vi "Read Pulsed Voltage.vi"(0 "VISA resource name":refnum<visa-resource-name>, 1 "Pulse Off Time (0.4 S)":dbl=0.4, 2 "Pulse On Time (0.2 S)":dbl=0.2, 5 "Source Measure Unit Channel (0: Channel A)":i32(ring) items=["Channel A", "Channel B"], 7 "Bias Level (0.001 A)":dbl=0.001, 9 "Pulse Level (1 A)":dbl=1.0, 11 "error in (no error)":errorcluster, 12 "Sweep Points (10)":i32=10) -> (4 "VISA resource name out":refnum<visa-resource-name>, 6 "Voltage (V)":dbl[](array[numeric]), 15 "error out":errorcluster)   [LabVIEW 2017, in "Keithley 2600 Series.lvlib"]
doc: "Performs a specified number of current pulse with a voltage measurement."
uses:
  <instrlib>/Keithley 2600 Series/Keithley 2600 Series.lvlib
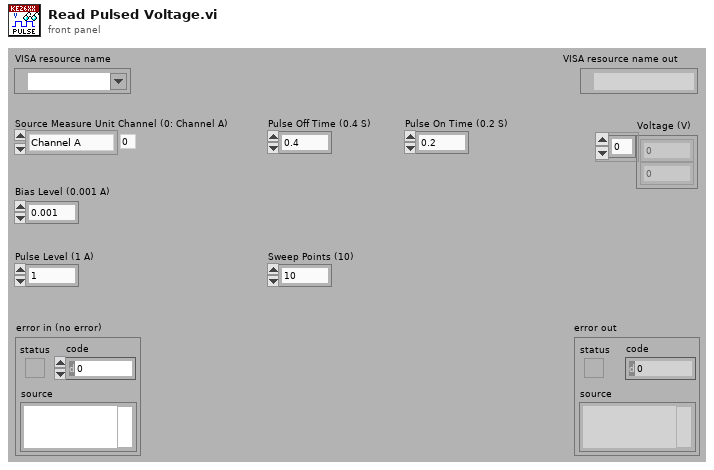
[diagram p1: front panel]
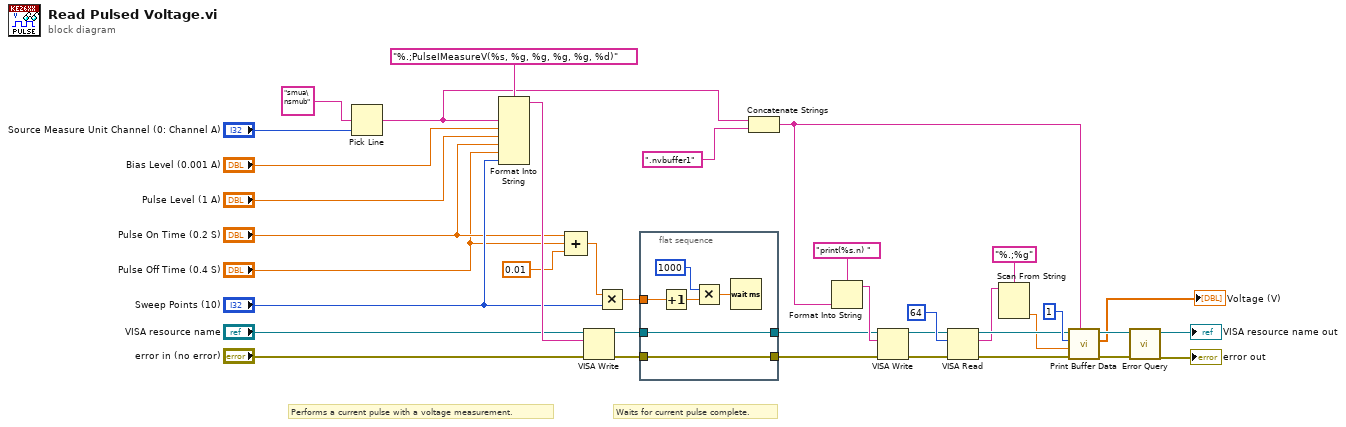
[diagram p0: block diagram]
diagram:
  # "Waits for current pulse complete."
  # "Performs a current pulse with a voltage measurement."
  n1 = Pick Line(multi-line string="smua\nsmub", line index="Source Measure Unit Channel (0: Channel A)") -> (output string=w7:string)  [unwired: 1 in]
  n2 = Format Into String(format string="%.;PulseIMeasureV(%s, %g, %g, %g, %g, %d)", w7, "Bias Level (0.001 A)", "Pulse Level (1 A)", "Pulse On Time (0.2 S)", "Pulse Off Time (0.4 S)", "Sweep Points (10)") -> (resulting string=w36:string)  [unwired: 2 in, 1 out]
  n3 = Compound Arithmetic op=ADD("Pulse On Time (0.2 S)", "Pulse Off Time (0.4 S)", 0.01 ("value")) -> (w20:dbl)
  n4 = VISA Write(VISA resource name="VISA resource name", write buffer=w36, error in (no error)="error in (no error)") -> (VISA resource name out=w27:refnum<visa-resource-name>, error out=w26:errorcluster)  [unwired: 1 out]
  n5 = Multiply(x=w20, y="Sweep Points (10)") -> (x*y=w24:dbl)
  n6 = flat-sequence {
    tunnel: w27 -> [w43]
    tunnel: w26 -> [w42]
    tunnel: [w43] -> w6
    tunnel: [w42] -> w5
    tunnel: w24 -> [w39]
    frame #0 {
      n7 = Increment(x=w39) -> (x+1=w38:dbl)
      n8 = Multiply(x=1000, y=w38) -> (x*y=w41:dbl)
      n9 = Wait (ms)(milliseconds to wait=w41) -> ()  [unwired: 1 out]
    }
  }
  n10 = Concatenate Strings(w7, ".nvbuffer1" ("string")) -> (w2:string)
  n11 = Format Into String(format string="print(%s.n) ", w2) -> (resulting string=w9:string)  [unwired: 2 in, 1 out]
  n12 = VISA Write(VISA resource name=w6, write buffer=w9, error in (no error)=w5) -> (VISA resource name out=w12:refnum<visa-resource-name>, error out=w11:errorcluster)  [unwired: 1 out]
  n13 = VISA Read(VISA resource name=w12, byte count=u32 64, error in (no error)=w11) -> (VISA resource name out=w17:refnum<visa-resource-name>, read buffer=w15:string, error out=w16:errorcluster)  [unwired: 1 out]
  n14 = Scan From String(format string="%.;%g", input string=w15) -> (output 1=w14:dbl)  [unwired: 3 in, 3 out]
  n15 = call <instrlib>:"Print Buffer Data.vi"("Reading Buffer (smua.nvbuffer1)"=w2, "error in (no error)"=w16, "End Index (1)"=w14, "Start Index (1)"=1 ("Start Index (0)"), "VISA resource name"=w17) -> ("error out"=w3:errorcluster, "Buffer Data"=→"Voltage (V)":dbl[], "VISA resource name out"=w4:refnum<visa-resource-name>)  [unwired: 4 in]
  n16 = call <instrlib>:"Error Query.vi"("error in (no error)"=w3, "VISA resource name"=w4) -> ("error out"=→"error out":errorcluster, "VISA resource name out"=→"VISA resource name out":refnum<visa-resource-name>)  [unwired: 6 in, 2 out]
